vi "gentec-SOLO-PE.Handle VISA Read Error.vi"(3 "error in":errorcluster) -> (0 "Timeout?":bool, 1 "error out":errorcluster)   [LabVIEW 2014, in "gentec-SOLO-PE - Driver.lvlib"]
uses:
  gentec-SOLO-PE - Driver.lvlib
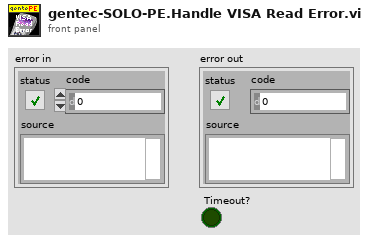
[diagram p1: front panel]
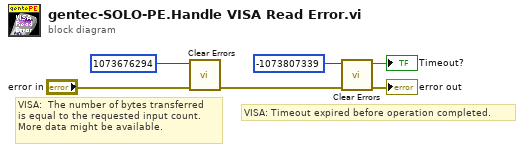
[diagram p0: block diagram]
diagram:
  # "VISA: Timeout expired before operation completed."
  # "VISA:  The number of bytes transferred\nis equal to the requested input count. \nMore data might be available."
  n1 = call <vilib>:"Clear Errors.vi"("error in (no error)"="error in", "specific error code to clear (0: all)"=1073676294) -> ("error out"=w5:errorcluster)  [unwired: 4 in, 1 out]
  n2 = call <vilib>:"Clear Errors.vi"("error in (no error)"=w5, "specific error code to clear (0: all)"=-1073807339) -> ("error out"=→"error out":errorcluster, "specific error cleared?"=→"Timeout?":bool)  [unwired: 4 in]
